vi "Init Hardware.vi"(8 "error in (no error)":errorcluster, 11 "DAQmx Digitizer in":refnum<class "DAQmx Digitizer.lvclass">) -> (0 "error out":errorcluster, 3 "DAQmx Digitizer out":refnum<class "DAQmx Digitizer.lvclass">)   [LabVIEW 2018, in "DAQmx Digitizer.lvclass"]
uses:
  DAQmx Digitizer.lvclass
  C:/github/NHMFL_Core/Libraries/Instruments/Pulse Driver/Pulse Driver.lvclass
  DAQmx Digitizer.lvclass/DAQmx Digitizer.ctl
  Instruments/Pulse Driver/Pulse Driver.lvclass/Pulse Driver.ctl
  Instruments/Pulse Driver/Read Pretrigger samples.vi
  Instruments/Pulse Driver/Read Samples per channel.vi
  Instruments/Pulse Driver/Write t0.vi
  Instruments/Pulse Driver/Write dt.vi
  Instruments/Pulse Driver/Write Set timing from UI.vi
  <vilib>/DAQmx/create/channels.llb/DAQmx Create Channel (AI-Voltage-Basic).vi
  <vilib>/DAQmx/configure/timing.llb/DAQmx Timing (Sample Clock).vi
  <vilib>/DAQmx/configure/trigger.llb/DAQmx Reference Trigger (Digital Edge).vi
  <vilib>/DAQmx/configure/events/hardwareSignals.llb/DAQmx Export Signal (Most Signals).vi
  <resource>/objmgr/daqmx.rc
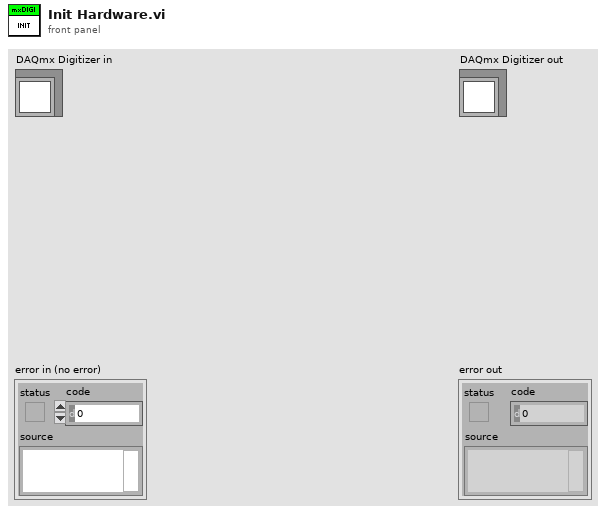
[diagram p1: front panel]
types:
  T1 = typedef "Pusle Driver Configuration.ctl" = cluster{"Pre-trigger duration":dbl, "Post-trigger duration":dbl, "Rate":dbl, "Ranges":dbl[], "Re-name channels":string[], "Active channels":string, "External clock":bool}
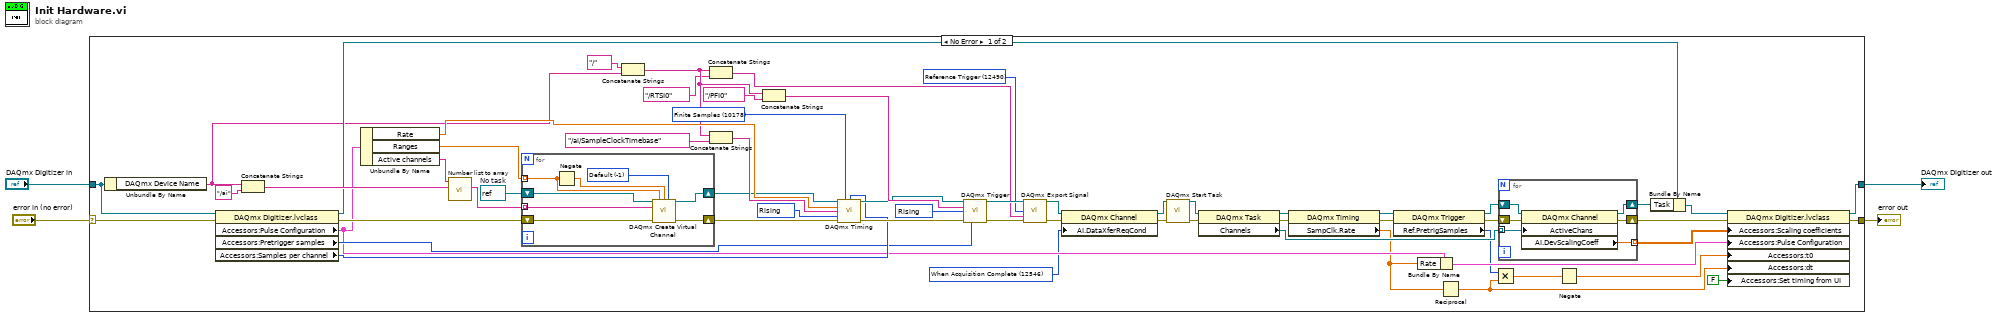
[diagram p0: block diagram]
diagram:
  n1 = case shown="No Error" "error in (no error)" {
    selector: "error in (no error)" -> [w44 w80]
    tunnel: [w45 w80] -> w3
    tunnel: [w46 w79] -> w1
    tunnel: "DAQmx Digitizer in" -> [w42 w79]
    frame No Error {
      w5 = 12546 items=["Onboard Memory More than Half Full"=10237, "Onboard Memory Not Empty"=10241, "Onboard Memory Custom Threshold"=12577, "When Acquisition Complete"=12546] ("AI.DataXferReqCond")
      w17 = 12490 items=["AI Convert Clock"=12484, "10MHz Reference Clock"=12536, "20MHz Timebase Clock"=12486, "Sample Clock"=12487, "Advance Trigger"=12488, "Reference Trigger"=12490, "Start Trigger"=12491, "Advance Complete Event"=12492, "AI Hold Complete Event"=12493, "Counter Output Event"=12494, "Change Detection Event"=12511, "Watchdog Timer Expired Event"=12512] ("signal")
      w49 = refnum<k21> refnum  # No task
      w56 = 10280 items=["Rising"=10280, "Falling"=10171] ("active edge")
      w57 = 10178 items=["Finite Samples"=10178, "Continuous Samples"=10123, "Hardware Timed Single Point"=12522] ("sample mode")
      w64 = 10280 items=["Rising"=10280, "Falling"=10171] ("edge")
      n2 = Unbundle By Name(w42) -> ("DAQmx Device Name"=w13:tag)
      n3 = property class="DAQmx Digitizer.lvclass"(reference=w42, error in=w44) -> (reference out=w41:refnum<class "DAQmx Digitizer.lvclass">, error out=w43:errorcluster, "Accessors:Pulse Configuration"=w33:T1, "Accessors:Pretrigger samples"=w34:u32, "Accessors:Samples per channel"=w35:i32)
      n4 = Concatenate Strings(w13, "/ai" ("string")) -> (w50:string)
      n5 = Unbundle By Name(w33) -> ("Rate"=w47:dbl, "Ranges"=w31:dbl[], "Active channels"=w52:string)
      n6 = call "Number list to array.vi"("Full names prefix"=w50, "Number list"=w52) -> ("Full names"=w48:string[])  [unwired: 8 in, 1 out]
      n7 = for {
        tunnel: w48 -> [w78] mode=indexing
        tunnel: w31 -> [w76] mode=indexing
        shift-right: [w73] -> w63
        shift-left: w43 -> [w77]
        shift-right: [w74] -> w29
        shift-left: w49 -> [w71]
        w72 = -1 items=["Default"=-1, "RSE"=10083, "NRSE"=10078, "Differential"=10106, "Pseudodifferential"=12529] ("input terminal configuration")
        n8 = Negate(x=w76) -> (-x=w75:dbl)
        n9 = call-poly <vilib>:"DAQmx Create Virtual Channel.vi"("task in"=w71, "maximum value"=w76, "minimum value"=w75, "input terminal configuration"=w72, "physical channels"=w78, "error in"=w77) -> ("task out"=w74:refnum<k21>, "error out"=w73:errorcluster)  [unwired: 8 in]
      }
      n10 = Concatenate Strings(tag "/" ("string"), w13) -> (w10:string)
      n11 = Concatenate Strings(w10, tag "/RTSI0" ("string")) -> (w11:string)
      n12 = Concatenate Strings(w10, tag "/ai/SampleClockTimebase" ("string")) -> (w55:string)
      n13 = Concatenate Strings(w10, tag "/PFI0" ("string")) -> (w61:string)
      n14 = call-poly <vilib>:"DAQmx Timing.vi"("task/channels in"=w29, "sample mode"=w57, "samples per channel"=w35, "rate"=w47, "source"=w55, "active edge"=w56, "error in"=w63) -> ("task out"=w59:refnum<k21>, "error out"=w60:errorcluster)  [unwired: 7 out]
      n15 = call-poly <vilib>:"DAQmx Trigger.vi"("task/channels in"=w59, "source"=w61, "edge"=w64, "error in"=w60, "pretrigger samples per channel"=w34) -> ("task out"=w18:refnum<k21>, "error out"=w16:errorcluster)  [unwired: 9 out]
      n16 = call-poly <vilib>:"DAQmx Export Signal.vi"("task/channels in"=w18, "signal"=w17, "output terminal"=w11, "error in"=w16) -> ("task out"=w7:refnum<k21>, "error out"=w15:errorcluster)  [unwired: 10 in]
      n17 = property class="DAQmx Channel"(reference=w7, error in=w15, "AI.DataXferReqCond"=w5) -> (reference out=w6:refnum<k21>, error out=w8:errorcluster)
      n18 = call <vilib>:"DAQmx Start Task.vi"("task/channels in"=w6, "error in"=w8) -> ("task out"=w54:refnum<k21>, "error out"=w53:errorcluster)  [unwired: 12 out]
      n19 = property class="DAQmx Task"(reference=w54, error in=w53) -> (reference out=w40:refnum<k21>, error out=w39:errorcluster, "Channels"=w30:refnum<k21>[])
      n20 = property class="DAQmx Timing"(reference=w40, error in=w39) -> (reference out=w27:refnum<k21>, error out=w24:errorcluster, "SampClk.Rate"=w28:dbl)
      n21 = property class="DAQmx Trigger"(reference=w27, error in=w24) -> (reference out=w26:refnum<k21>, error out=w25:errorcluster, "Ref.PretrigSamples"=w23:u32)
      n22 = Bundle By Name(cluster=w33, "Rate"=w28) -> (w32:T1)
      n23 = Reciprocal(x=w28) -> (1/x=w22:dbl)
      n24 = Multiply(x=w23, y=w22) -> (x*y=w21:dbl)
      n25 = for {
        tunnel: w30 -> [w70] mode=indexing
        shift-right: [w67] -> w38
        shift-left: w26 -> [w68]
        shift-right: [w66] -> w37
        shift-left: w25 -> [w69]
        tunnel: [w65] -> w36 mode=indexing
        n26 = property class="DAQmx Channel"(reference=w68, error in=w69, "ActiveChans"=w70) -> (reference out=w67:refnum<k21>, error out=w66:errorcluster, "AI.DevScalingCoeff"=w65:dbl[])
      }
      n27 = Negate(x=w21) -> (-x=w19:dbl)
      n28 = Bundle By Name(cluster=w41, "Task"=w38) -> (w62:refnum<class "DAQmx Digitizer.lvclass">)
      n29 = property class="DAQmx Digitizer.lvclass"(reference=w62, error in=w37, "Accessors:Scaling coefficients"=w36, "Accessors:Pulse Configuration"=w32, "Accessors:t0"=w19, "Accessors:dt"=w22, "Accessors:Set timing from UI"=FALSE ("Set timing from UI")) -> (reference out=w46:refnum<class "DAQmx Digitizer.lvclass">, error out=w45:errorcluster)
    }
    frame Error {
    }
  }
  "error out" <- w3
  "DAQmx Digitizer out" <- w1
